vi "picoG Main.vi"(11 "Ready Notifier":refnum<notifier>) -> ()   [LabVIEW 2020, in "PicoG-App.lvlib"]
uses:
  PicoG-App.lvlib
  picoG/picoG.lvclass
panel:
  # "This VI can be run from the development environment to start the app. When run this way it will remain visible. When run via the executable's splash UI it will not be visible."
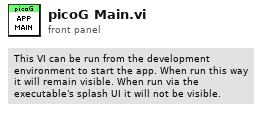
[diagram p1: front panel]
types:
  T1 = enum32{"invalid app kind", "Development System", "Run Time System", "Student Edition", "Embedded LabVIEW", "Evaluation", "Custom"}
  T2 = enum32{"Invalid", "Standard", "Closed", "Hidden", "Minimized", "Maximized"}
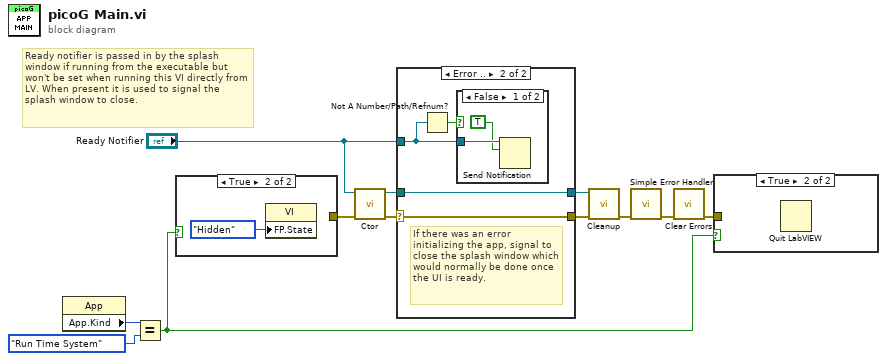
[diagram p0: block diagram]
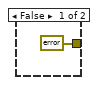
[diagram p2: hidden frame]
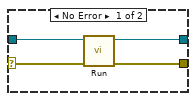
[diagram p3: hidden frame]
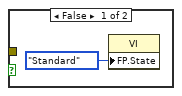
[diagram p5: hidden frame]
diagram:
  # "Ready notifier is passed in by the splash window if running from the executable but won't be set when running this VI directly from LV. When present it is used to signal the splash window to close."
  n1 = property class="App"() -> ("App.Kind"=w12:T1)  [unwired: 2 in, 2 out]
  n2 = Equal?(x=w12, y=T1."Run Time System" ("Application:Kind")) -> (x = y?=w1:bool)
  n3 = case shown="True" w1 {
    tunnel: [errorcluster {"status"=FALSE, "code"=0, "source"=""} ("error out") _] -> w3
    frame False {
    }
    frame True {
      n4 = property class="VI"("FP.State"=T2."Hidden" ("Front Panel Window:State")) -> ()  [unwired: 2 in, 2 out]
    }
  }
  n5 = call "Ctor.vi"("error in (no error)"=w3, "Ready Notifier"="Ready Notifier") -> ("error out"=w9:errorcluster, "picoG out"=w8:refnum<class "picoG.lvclass">)  [unwired: 8 in]
  n6 = case shown="Error .." w9 {
    selector: w9 -> [w15 w19]
    tunnel: "Ready Notifier" -> [_ w21]
    tunnel: w8 -> [w18 w20]
    tunnel: [w17 w19] -> w6
    tunnel: [w16 w20] -> w7
    frame No Error {
      n7 = call "Run.vi"("error in (no error)"=w15, "picoG in"=w18) -> ("error out"=w17:errorcluster, "picoG out"=w16:refnum<class "picoG.lvclass">)  [unwired: 8 in]
    }
    frame Error {
      # "If there was an error initializing the app, signal to close the splash window which would normally be done once the UI is ready."
      n8 = Not A Number/Path/Refnum?(number/path/refnum=w21) -> (NaN/Path/Refnum?=w22:bool)
      n9 = case shown="False" w22 {
        tunnel: w21 -> [w24 _]
        frame False {
          n10 = Send Notification(notification=TRUE, notifier=w24) -> ()  [unwired: 1 in, 2 out]
        }
        frame True {
        }
      }
    }
  }
  n11 = call "Cleanup.vi"("error in (no error)"=w6, "picoG in"=w7) -> ("error out"=w5:errorcluster)  [unwired: 9 in]
  n12 = call <vilib>:"Simple Error Handler.vi"("error in (no error)"=w5) -> ("error out"=w4:errorcluster)  [unwired: 4 in, 4 out]
  n13 = call <vilib>:"Clear Errors.vi"("error in (no error)"=w4) -> ("error out"=w2:errorcluster)  [unwired: 5 in, 1 out]
  n14 = case shown="True" w1 {
    tunnel: w2 -> [_ _]
    frame False {
      n15 = property class="VI"("FP.State"=T2."Standard" ("Front Panel Window:State")) -> ()  [unwired: 2 in, 2 out]
    }
    frame True {
      n16 = Quit LabVIEW() -> ()  [unwired: 1 in]
    }
  }
